vi "Day 4.vi"() -> ()   [LabVIEW 2019]
panel:
  out "Guard, Minute (Most Slept Minute)":string
  out "Amount of Times Sleeping During Most Slept Minute":i32
  out "Guard Who Sleeps Most, Minute Most Slept":string
  out "Number of Times Slept at Minute Most Slept":i32
  out "Total Minutes Slept":i32
  out "Guard Who Sleeps Most":string
  out "Error Out":errorcluster
  in  "Example Input":string="[1518-11-01 00:00] Guard #10 begins shift\n[1518-11-01 00:05] falls asleep\n[1518-11-01 00:25] wakes up\n[1518-11-01 00:30] falls asleep\n[1518-11-01 00:55] wakes up\n[1518-11-01 23:58] Guard #99 begins shift\n[1518-11-02 00:40] falls asleep\n[1518-11-02 00:50] wakes up\n[1518-11-03 00:05] Guard #10 begins shift\n[1518-11-03 00:24] falls asleep\n[1518-11-03 00:29] wakes up\n[1518-11-04 00:02] Guard #99 begins shift\n[1518-11-04 00:36] falls asleep\n[1518-11-04 00:46] wakes up\n[1518-11-05 00:03] Guard #99 begins shift\n[1518-11-05 00:45] falls asleep\n[1518-11-05 00:55] wakes up"
  in  "Use Example Input":bool
  in  "Error In":errorcluster
  in  "Relative Path to Input File":string="Day 4\\Day 4 Raw Input.txt"
  # "Part 1"
  # "Part 2"
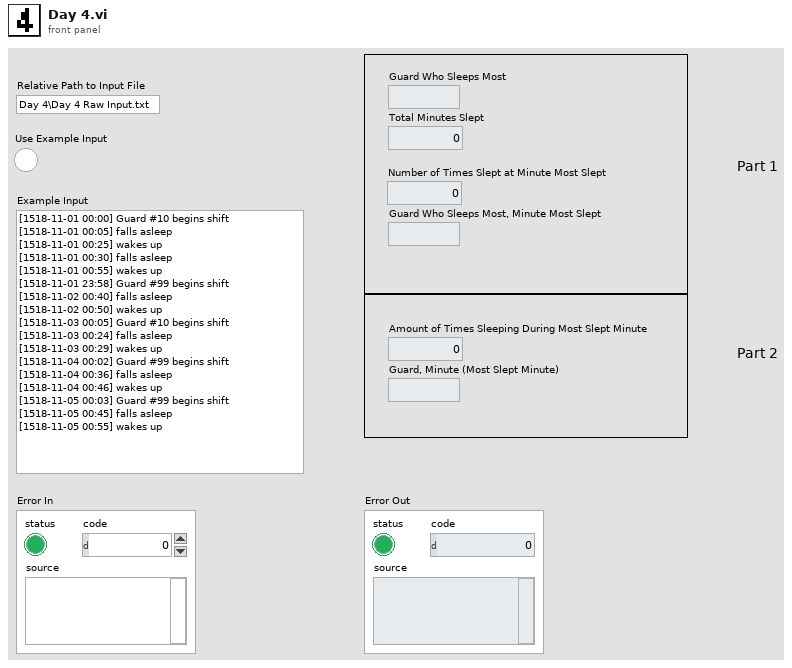
[diagram p1: front panel]
types:
  T1 = typedef "Log Entry.ctl" = cluster{"Guard Sleep Minutes":map{string, i32}, "Guard Total Sleep":map{string, i32}, "Time Fell Asleep":timestamp, "Guard #":i32}
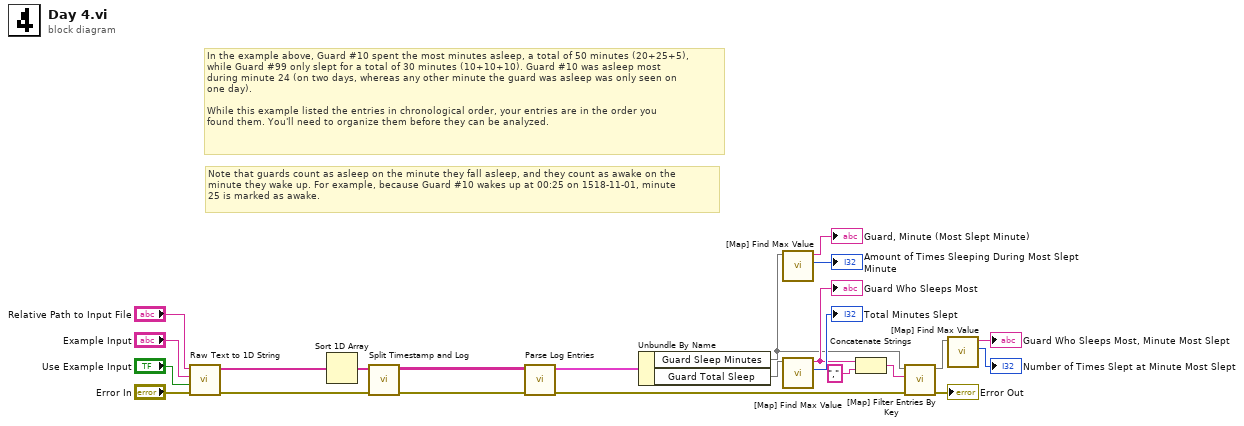
[diagram p0: block diagram]
diagram:
  # "In the example above, Guard #10 spent the most minutes asleep, a total of 50 minutes (20+25+5), \nwhile Guard #99 only slept for a total of 30 minutes (10+10+10). Guard #10 was asleep most \nduring minute 24 (on two days, whereas any other minute the guard was asleep was only seen on \none day).\n\nWhile this example listed the entries in chronological order, your entries are in the order you \nfound them. You'll need to organize them before they can be analyzed."
  # "Note that guards count as asleep on the minute they fall asleep, and they count as awake on the \nminute they wake up. For example, because Guard #10 wakes up at 00:25 on 1518-11-01, minute \n25 is marked as awake."
  n1 = call "Raw Text to 1D String.vi"("Error In"="Error In", "Use Example Input"="Use Example Input", "Example Input"="Example Input", "Relative Path to Input File"="Relative Path to Input File") -> ("Error Out"=w15:errorcluster, "1D String Array"=w21:string[])  [unwired: 6 in]
  n2 = Sort 1D Array(array=w21) -> (sorted array=w20:string[])
  n3 = call "Split Timestamp and Log.vi"("error in (no error)"=w15, "Array"=w20) -> ("error out"=w16:errorcluster, "Split String"=w17:string[][])  [unwired: 8 in]
  n4 = call "Parse Log Entries.vi"("error in (no error)"=w16, "Split String"=w17) -> ("error out"=w14:errorcluster, "Day 4 Data"=w3:T1)  [unwired: 8 in]
  n5 = Unbundle By Name(w3) -> ("Guard Sleep Minutes"=w1:map{string, i32}, "Guard Total Sleep"=w2:map{string, i32})
  n6 = call "[Map] Find Max Value.vi"("Map"=w1) -> ("Max Value"=→"Amount of Times Sleeping During Most Slept Minute":i32, "Key With Max Value"=→"Guard, Minute (Most Slept Minute)":string)  [unwired: 9 in]
  n7 = call "[Map] Find Max Value.vi"("Map"=w2) -> ("Max Value"=→"Total Minutes Slept":i32, "Key With Max Value"=w10:string)  [unwired: 9 in]
  "Guard Who Sleeps Most" <- w10
  n8 = Concatenate Strings(w10, "," ("string")) -> (w12:string)
  n9 = call "[Map] Filter Entries By Key.vi"("error in (no error)"=w14, "Key Filter"=w12, "Map in"=w1) -> ("Error Out"=→"Error Out":errorcluster, "Map out"=w9:map{string, i32})  [unwired: 7 in]
  n10 = call "[Map] Find Max Value.vi"("Map"=w9) -> ("Max Value"=→"Number of Times Slept at Minute Most Slept":i32, "Key With Max Value"=→"Guard Who Sleeps Most, Minute Most Slept":string)  [unwired: 9 in]
